vi "nmap.vi"(3 "error in (no error)":errorcluster) -> (0 "error out":errorcluster, 2 "IPs":string[](array[string]))   [LabVIEW 2013]
panel:
  in  "command line":string="nmap -sP -n -T5 192.168.10.1-254"
  out "size(s)":i32
  out "array":string[](array[string])
  out "standard output":string
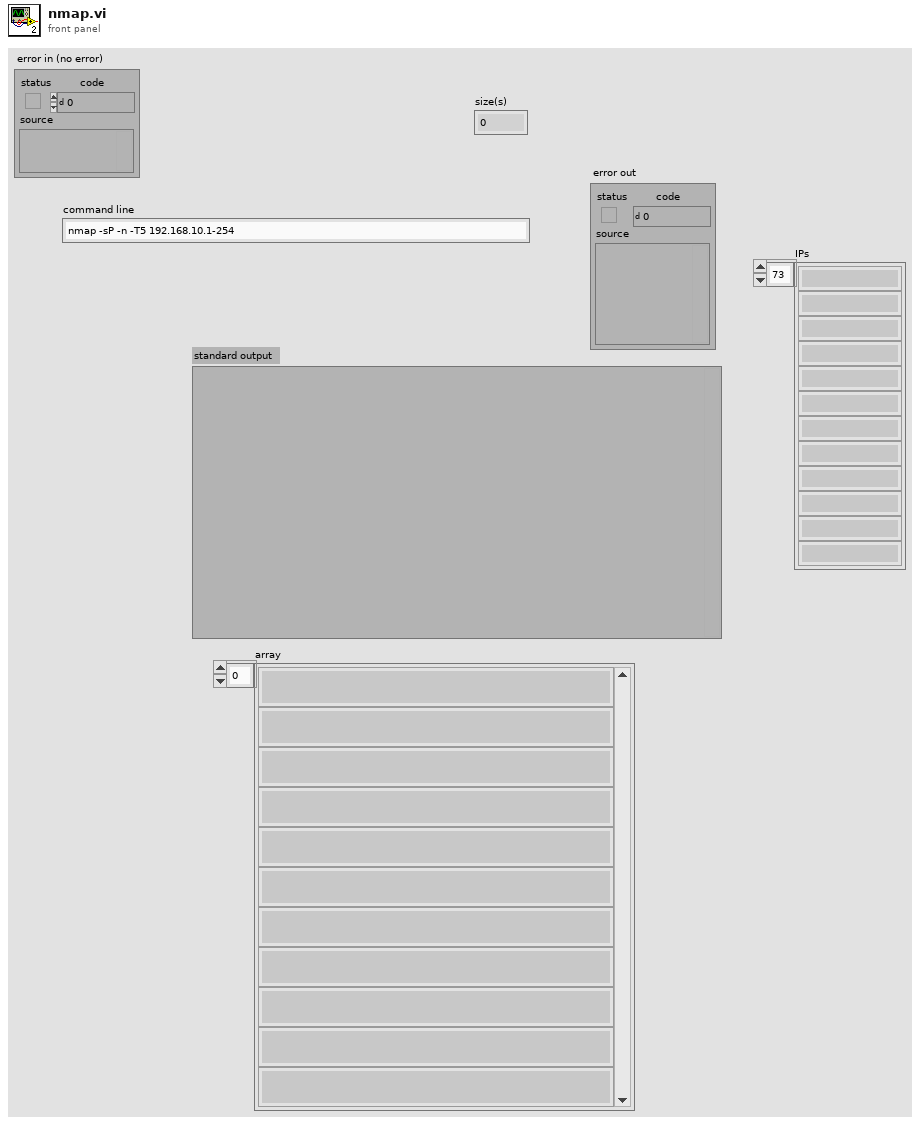
[diagram p1: front panel]
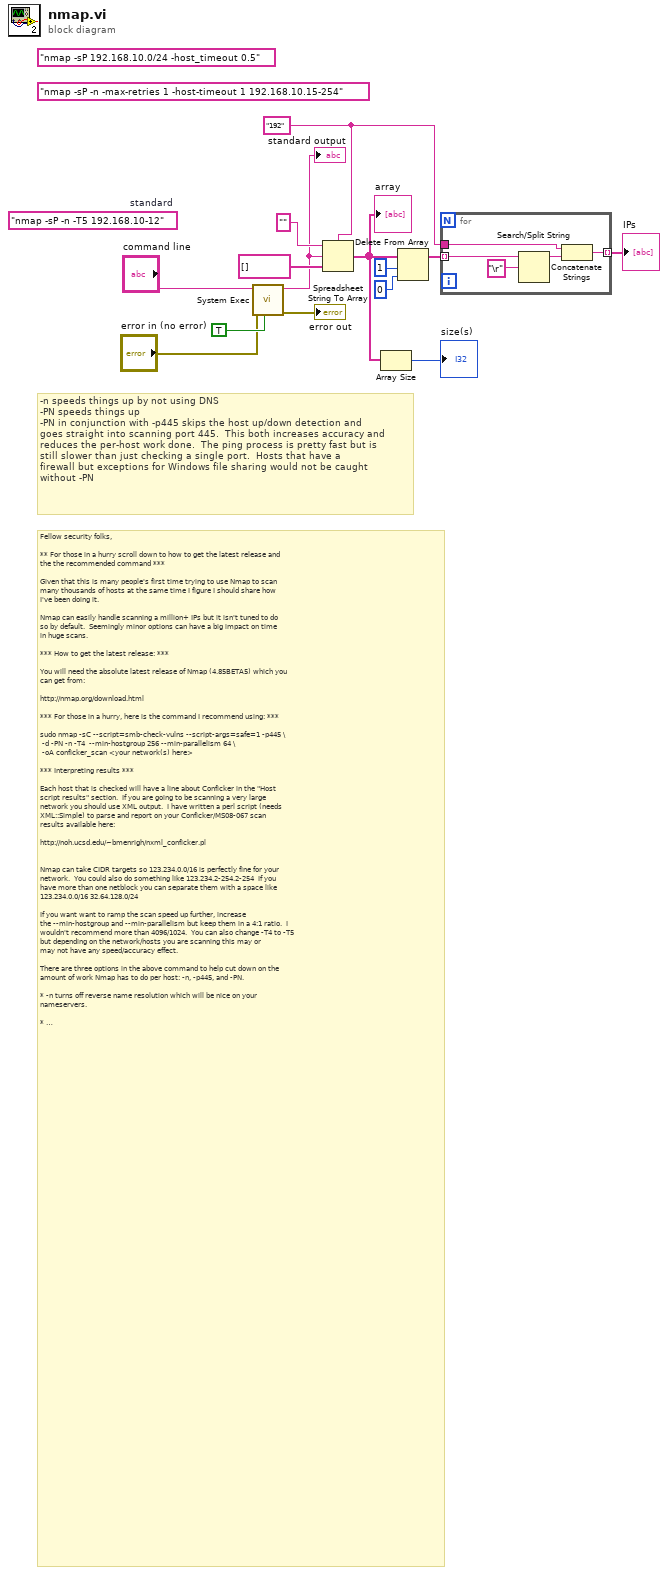
[diagram p0: block diagram]
diagram:
  (unwired) "nmap -sP -n -T5 192.168.10-12"  # standard
  (unwired) "nmap -sP -n -max-retries 1 -host-timeout 1 192.168.10.15-254" ("command line")
  w2 = "192" ("spreadsheet string")
  (unwired) "nmap -sP 192.168.10.0/24 -host_timeout 0.5" ("command line")
  # "Fellow security folks,\n\n** For those in a hurry scroll down to how to get the latest release and\nthe the recommended command ***\n\nGiven that this is many people's first time trying to use Nmap to scan\nmany thousands of hosts at the same time I figure I should share how\nI've been doing it.\n\nNmap can easily handle scanning a million+ IPs but it isn't tuned to do\nso by default.  Seemingly minor options can have a big impact on time\nin huge scans.\n\n*** How to get the latest release: ***\n\nYou will need the absolute latest release of Nmap (4.85BETA5) which you\ncan get from:\n\nhttp://nmap.org/download.html\n\n*** For those in a hurry, here is the command I recommend using: ***\n\nsudo nmap -sC --script=smb-check-vulns --script-args=safe=1 -p445 \\\n -d -PN -n -T4  --min-hostgroup 256 --min-parallelism 64 \\\n -oA conficker_scan <your network(s) here>\n\n*** Interpreting results ***\n\nEach host that is checked will have a line about Conficker in the \"Host\nscript results\" section.  If you are going to be scanning a very large\nnetwork you should use XML output.  I have written a perl script (needs\nXML::Simple) to parse and report on your Conficker/MS08-067 scan\nresults available here:\n\nhttp://noh.ucsd.edu/~bmenrigh/nxml_conficker.pl\n\n\nNmap can take CIDR targets so 123.234.0.0/16 is perfectly fine for your\nnetwork.  You could also do something like 123.234.2-254.2-254  If you\nhave more than one netblock you can separate them with a space like\n123.234.0.0/16 32.64.128.0/24\n\nIf you want want to ramp the scan speed up further, increase\nthe --min-hostgroup and --min-parallelism but keep them in a 4:1 ratio.  I\nwouldn't recommend more than 4096/1024.  You can also change -T4 to -T5\nbut depending on the network/hosts you are scanning this may or\nmay not have any speed/accuracy effect.\n\nThere are three options in the above command to help cut down on the\namount of work Nmap has to do per host: -n, -p445, and -PN.\n\n* -n turns off reverse name resolution which will be nice on your\nnameservers.\n\n* -PN in conjunction with -p445 skips the host up/down detection and\ngoes straight into scanning port 445.  This both increases accuracy and\nreduces the per-host work done.  The ping process is pretty fast but is\nstill slower than just checking a single port.  Hosts that have a\nfirewall but exceptions for Windows file sharing would not be caught\nwithout -PN.\n\nIt is important to note that scanning for Conficker has the small\nchance of crashing an unpatched host.  Patched and infected hosts won't\nbe crashed though.  Note that if Conficker scans unpatched hosts they\nare even more likely to crash than with this check so the benefits\nprobably outweigh the drawbacks.\n\nIf you have questions about this script/using Nmap drop a note to\nnmap-dev () insecure org"
  # "-n speeds things up by not using DNS\n-PN speeds things up\n-PN in conjunction with -p445 skips the host up/down detection and\ngoes straight into scanning port 445.  This both increases accuracy and\nreduces the per-host work done.  The ping process is pretty fast but is\nstill slower than just checking a single port.  Hosts that have a\nfirewall but exceptions for Windows file sharing would not be caught\nwithout -PN"
  n1 = call <vilib>:"System Exec.vi"("run minimized? (F)"=TRUE, "error in (no error)"="error in (no error)", "command line"="command line") -> ("error out"=→"error out":errorcluster, "standard output"=w8:string)  [unwired: 5 in, 2 out]
  "standard output" <- w8
  n2 = Spreadsheet String To Array(delimiter (Tab)=w2, format string="", spreadsheet string=w8, array type (2D Dbl)=string[] []) -> (array=w7:string[])
  "array" <- w7
  n3 = Array Size(array=w7) -> (size(s)=→"size(s)":i32)
  n4 = Delete From Array(array=w7, length=1, index=0) -> (array with subset deleted=w4:string[])  [unwired: 1 out]
  n5 = for {
    tunnel: w4 -> [w19] mode=indexing
    tunnel: [w17] -> w3 mode=indexing
    tunnel: w2 -> [w16]
    n6 = Search/Split String(string=w19, search string/char (-)="\r") -> (substring before match=w15:string)  [unwired: 1 in, 2 out]
    n7 = Concatenate Strings(w16, w15) -> (w17:string)
  }
  "IPs" <- w3
